vi "HexOrDecimalStringComparison.vi"(6 "Comparison Type":T1(ring)=enum."Equal (==)", 7 "Hex Conv For Input String?":bool=TRUE, 9 "High Comparison (LEGE & GELE Only)":string, 10 "Low Comparison (Use Default)":string, 11 "Input":string) -> (2 "Pass/Fail?":bool, 3 "Converted Input":u32)   [LabVIEW 2016]
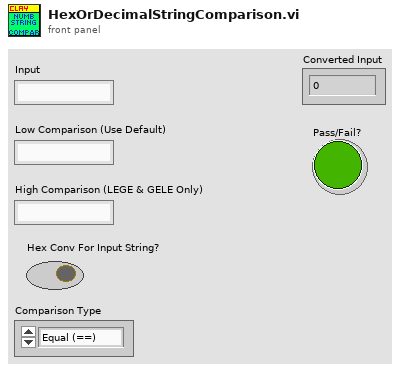
[diagram p1: front panel]
types:
  T1 = enum16{"LEGE  (<=Low OR >=High", "GELE (>= Low && <=High)", "Less than or Equal (<=)", "String Remove All Spaces.viGreater than or Equal (>=)", "Not Equal (!=)", "Equal (==)", "Less Than (<)", "Greater Than (>)"}
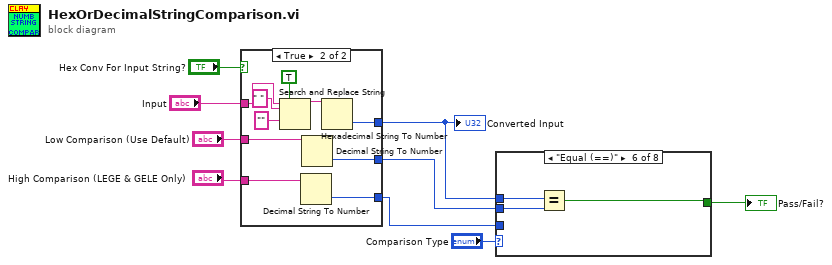
[diagram p0: block diagram]
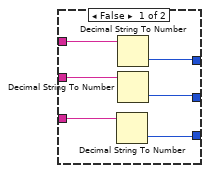
[diagram p2: hidden frame]
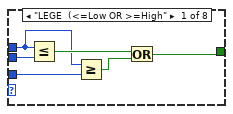
[diagram p3: hidden frame]
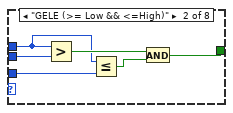
[diagram p4: hidden frame]
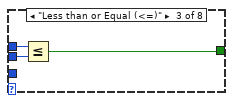
[diagram p5: hidden frame]
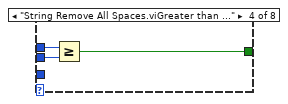
[diagram p6: hidden frame]
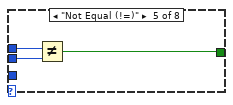
[diagram p7: hidden frame]
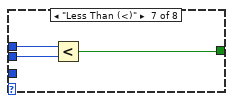
[diagram p8: hidden frame]
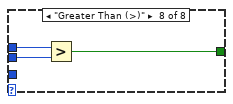
[diagram p9: hidden frame]
diagram:
  n1 = case shown="True" "Hex Conv For Input String?" {
    tunnel: "Input" -> [w11 w23]
    tunnel: "Low Comparison (Use Default)" -> [w13 w21]
    tunnel: "High Comparison (LEGE & GELE Only)" -> [w15 w20]
    tunnel: [w12 w19] -> w2
    tunnel: [w10 w18] -> w3
    tunnel: [w14 w17] -> w1
    frame False {
      n2 = Decimal String To Number(string=w15) -> (number=w14:i32)  [unwired: 2 in, 1 out]
      n3 = Decimal String To Number(string=w11) -> (number=w10:i32)  [unwired: 2 in, 1 out]
      n4 = Decimal String To Number(string=w13) -> (number=w12:i32)  [unwired: 2 in, 1 out]
    }
    frame True {
      n5 = Search and Replace String(replace all?=TRUE ("replace all? (F)"), input string=w23, search string=" ", replace string="" ("replace string (\"\")")) -> (result string=w22:string)  [unwired: 4 in, 3 out]
      n6 = Decimal String To Number(string=w20) -> (number=w17:i32)  [unwired: 2 in, 1 out]
      n7 = Decimal String To Number(string=w21) -> (number=w19:i32)  [unwired: 2 in, 1 out]
      n8 = Hexadecimal String To Number(string=w22) -> (number=w18:u32)  [unwired: 2 in, 1 out]
    }
  }
  "Converted Input" <- w3
  n9 = case shown="\"Equal (==)\"" "Comparison Type" {
    tunnel: [w29 w35 w40 w43 w46 w49 w52 w55] -> w5
    tunnel: w3 -> [w27 w32 w39 w42 w45 w48 w51 w54]
    tunnel: w2 -> [w28 w34 w38 w41 w44 w47 w50 w53]
    tunnel: w1 -> [w26 w33 _ _ _ _ _ _]
    frame "LEGE  (<=Low OR >=High" {
      n10 = Less Or Equal?(x=w27, y=w28) -> (x <= y?=w31:bool)
      n11 = Greater Or Equal?(x=w27, y=w26) -> (x >= y?=w30:bool)
      n12 = Or(x=w31, y=w30) -> (x .or. y?=w29:bool)
    }
    frame "GELE (>= Low && <=High)" {
      n13 = Greater?(x=w32, y=w34) -> (0:w36:bool)
      n14 = Less Or Equal?(x=w32, y=w33) -> (x <= y?=w37:bool)
      n15 = And(x=w36, y=w37) -> (x .and. y?=w35:bool)
    }
    frame "Less than or Equal (<=)" {
      n16 = Less Or Equal?(x=w39, y=w38) -> (x <= y?=w40:bool)
    }
    frame "String Remove All Spaces.viGreater than or Equal (>=)" {
      n17 = Greater Or Equal?(x=w42, y=w41) -> (x >= y?=w43:bool)
    }
    frame "Not Equal (!=)" {
      n18 = Not Equal?(x=w45, y=w44) -> (x != y?=w46:bool)
    }
    frame "Equal (==)" {
      n19 = Equal?(x=w48, y=w47) -> (x = y?=w49:bool)
    }
    frame "Less Than (<)" {
      n20 = Less?(x=w51, y=w50) -> (x < y?=w52:bool)
    }
    frame "Greater Than (>)" {
      n21 = Greater?(x=w54, y=w53) -> (0:w55:bool)
    }
  }
  "Pass/Fail?" <- w5
